vi "Write outgoing label data.vi"(4 "ScheduledSDI":bool, 6 "Iteration":i32, 8 "error in (no error)":errorcluster, 10 "Values":dbl[](array[numeric]), 11 "Driver Data":T1 {"Num Bits" min=1 max=32; "Start Bit" min=8 max=31}) -> (0 "error out":errorcluster)   [LabVIEW 2011, in "AIT 1553 Custom Device.lvlib"]
uses:
  AIT 1553 Custom Device.lvlib
  RT Controls/Driver Data.ctl
  Controls and Global/Start Bit.ctl
  Controls and Global/Number of Bits.ctl
  <instrlib>/AIT 429/AIT 429.lvlib
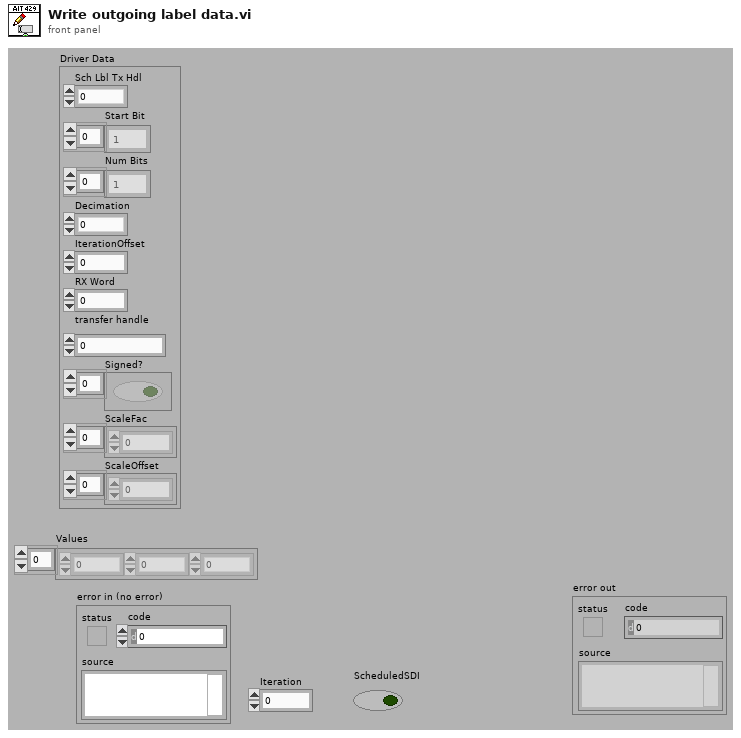
[diagram p1: front panel]
types:
  T1 = typedef "AIT 1553 Custom Device.lvlib/Driver Data.ctl" = cluster{"Sch Lbl Tx Hdl":u32, "Start Bit":T2[], "Num Bits":T3[], "Decimation":i32, "IterationOffset":i32, "RX Word":u32, "transfer handle":u32, "Signed?":bool[], "ScaleFac":dbl[], "ScaleOffset":dbl[]}
  T2 = typedef "AIT 1553 Custom Device.lvlib/Start Bit.ctl" = i32
  T3 = typedef "AIT 1553 Custom Device.lvlib/Number of Bits.ctl" = i32
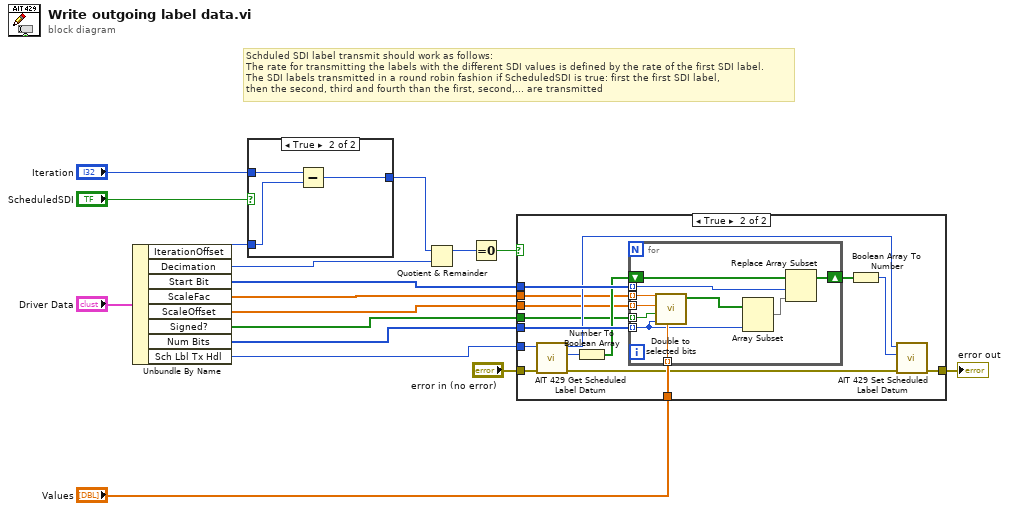
[diagram p0: block diagram]
diagram:
  # "Schduled SDI label transmit should work as follows:\nThe rate for transmitting the labels with the different SDI values is defined by the rate of the first SDI label.\nThe SDI labels transmitted in a round robin fashion if ScheduledSDI is true: first the first SDI label, \nthen the second, third and fourth than the first, second,... are transmitted"
  n1 = Unbundle By Name("Driver Data") -> ("IterationOffset"=w2:i32, "Decimation"=w16:i32, "Start Bit"=w13:T2[], "ScaleFac"=w7:dbl[], "ScaleOffset"=w6:dbl[], "Signed?"=w5:bool[], "Num Bits"=w12:T3[], "Sch Lbl Tx Hdl"=w8:u32)
  n2 = case shown="True" "ScheduledSDI" {
    tunnel: "Iteration" -> [w18 w19]
    tunnel: [w18 w21] -> w3
    tunnel: w2 -> [_ w20]
    frame False {
    }
    frame True {
      n3 = Subtract(x=w19, y=w20) -> (x-y=w21:i32)
    }
  }
  n4 = Quotient & Remainder(x=w3, y=w16) -> (x-y*floor(x/y)=w15:i32)  [unwired: 1 out]
  n5 = Equal To 0?(x=w15) -> (x = 0?=w14:bool)
  n6 = case shown="True" w14 {
    tunnel: w13 -> [_ w37]
    tunnel: w12 -> [_ w36]
    tunnel: "Values" -> [_ w35]
    tunnel: "error in (no error)" -> [w22 w33]
    tunnel: [w22 w34] -> w9
    tunnel: w8 -> [_ w32]
    tunnel: w7 -> [_ w25]
    tunnel: w6 -> [_ w24]
    tunnel: w5 -> [_ w23]
    frame False {
    }
    frame True {
      n7 = call <instrlib>:"AIT 429 Get Scheduled Label Datum.vi"("error in (no error)"=w33, "scheduled label handle"=w32) -> ("error out"=w28:errorcluster, "data word"=w30:u32, "scheduled label handle"=w31:u32)  [unwired: 7 in]
      n8 = Number To Boolean Array(number=w30) -> (Boolean array=w29:bool[])
      n9 = for {
        tunnel: w37 -> [w46] mode=indexing
        tunnel: w36 -> [w41] mode=indexing
        tunnel: w35 -> [w42] mode=indexing
        shift-right: [w44] -> w27
        shift-left: w29 -> [w47]
        tunnel: w25 -> [w40] mode=indexing
        tunnel: w24 -> [w39] mode=indexing
        tunnel: w23 -> [w38] mode=indexing
        n10 = call "Double to selected bits.vi"("Double"=w42, "Number of Bits"=w41, "Signed?"=w38, "ScaleOffset"=w39, "ScaleFac"=w40) -> ("Bits"=w43:bool[])  [unwired: 6 in]
        n11 = Array Subset(array=w43, length=w41) -> (w45:bool[])  [unwired: 1 in]
        n12 = Replace Array Subset(array=w47, new element=w45, index=w46) -> (w44:bool[])
      }
      n13 = Boolean Array To Number(Boolean array=w27) -> (number=w26:u32)
      n14 = call <instrlib>:"AIT 429 Set Scheduled Label Datum.vi"("error in (no error)"=w28, "word"=w26, "scheduled label handle"=w31) -> ("error out"=w34:errorcluster)  [unwired: 7 in, 1 out]
    }
  }
  "error out" <- w9
